vi "Istwerte verarbeiten Regler.vi"(8 "error in (no error)":errorcluster caption="Fehler (Eingang, kein Fehler)", 9 "Index":u16, 10 "Istwerte":u16[](array[numeric]), 11 "mini8 Steuerung PNS Eingang":refnum<class "mini8 Steuerung PNS.lvclass">) -> (0 "error out":errorcluster caption="Fehler (Ausgang)", 3 "mini8 Steuerung PNS Ausgang":refnum<class "mini8 Steuerung PNS.lvclass">)   [LabVIEW 2020, in "mini8 Steuerung PNS.lvclass"]
uses:
  mini8 Steuerung PNS.lvclass
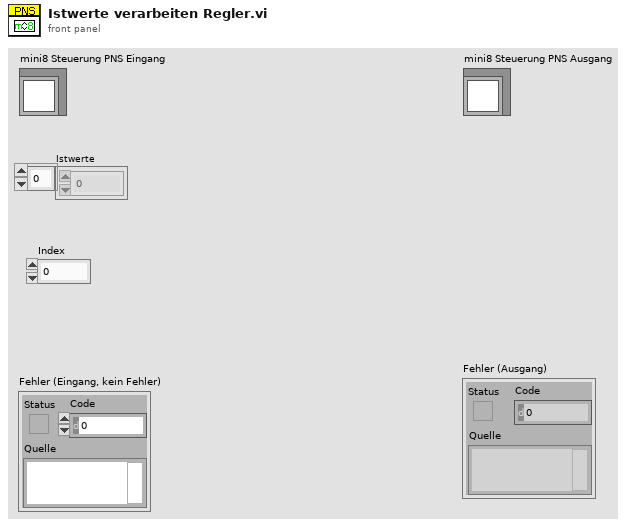
[diagram p1: front panel]
types:
  T1 = typedef "Steuerung PNS.lvclass/Regler.ctl" = cluster{"Istwert":i16, "Sollwert":i16, "Alarm MIN":i16, "Alarm MAX":i16, "Regler sperren":i16, "Analog Ausgang":i16}[]
  T2 = cluster{"Istwerte[0]":u16, "Istwerte[1]":u16, "Istwerte[2]":u16, "Istwerte[3]":u16, "Istwerte[4]":u16, "Istwerte[5]":u16}
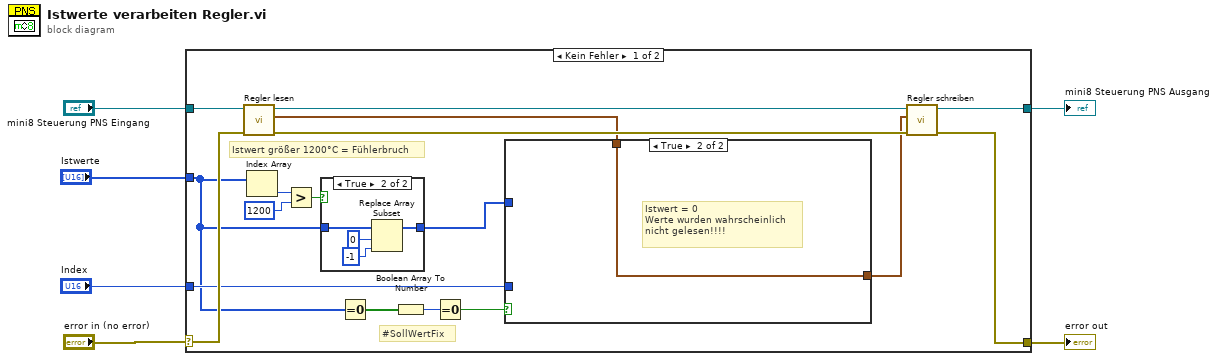
[diagram p0: block diagram]
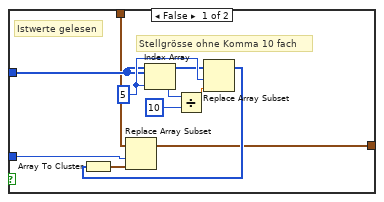
[diagram p2: hidden frame]
diagram:
  n1 = case shown="Kein Fehler" "error in (no error)" {
    selector: "error in (no error)" -> [w15 w41]
    tunnel: [w14 w41] -> w5
    tunnel: [w17 w40] -> w3
    tunnel: "mini8 Steuerung PNS Eingang" -> [w23 w40]
    tunnel: "Istwerte" -> [w9 _]
    tunnel: "Index" -> [w11 _]
    frame No Error {
      # "#SollWertFix"
      # "Istwert größer 1200°C = Fühlerbruch"
      n2 = call-dynamic "Regler lesen.vi"("error in (no error)"=w15, "Steuerung PNS (Eingang)"=w23) -> ("error out"=w16:errorcluster, "Regler"=w12:T1, "Steuerung PNS (Ausgang)"=w18:refnum<class "mini8 Steuerung PNS.lvclass">)  [unwired: 7 in]
      n3 = Index Array(array=w9) -> (element=w20:u16)  [unwired: 1 in]
      n4 = Greater?(x=w20, y=i16 1200) -> (0:w21:bool)
      n5 = case shown="True" w21 {
        tunnel: w9 -> [w35 w36]
        tunnel: [w35 w39] -> w13
        frame False {
        }
        frame True {
          n6 = Replace Array Subset(array=w36, new element=i16 -1 ("Neues Element/Teil-Array"), index=0 ("Index")) -> (w39:u16[])
        }
      }
      n7 = Equal To 0?(x=w9) -> (x = 0?=w8:bool[])
      n8 = Boolean Array To Number(Boolean array=w8) -> (number=w7:u32)
      n9 = Equal To 0?(x=w7) -> (x = 0?=w19:bool)
      n10 = case shown="True" w19 {
        tunnel: w13 -> [w28 _]
        tunnel: w12 -> [w27 w34]
        tunnel: w11 -> [w25 _]
        tunnel: [w24 w34] -> w10
        frame False {
          w33 = 5 ("Index")
          # "Istwerte gelesen"
          # "Stellgrösse ohne Komma 10 fach"
          n11 = Index Array(array=w28, index=w33) -> (element=w32:u16)
          n12 = Divide(x=w32, y=i16 10) -> (x/y=w30:dbl)
          n13 = Replace Array Subset(array=w28, new element=w30, index=w33) -> (w26:u16[])
          n14 = Array To Cluster(array=w26) -> (cluster=w29:T2)
          n15 = Replace Array Subset(array=w27, new element=w29, index=w25) -> (w24:T1)
        }
        frame True {
          # "Istwert = 0\nWerte wurden wahrscheinlich\nnicht gelesen!!!!"
        }
      }
      n16 = call-dynamic "Regler schreiben.vi"("error in (no error)"=w16, "Regler"=w10, "Steuerung PNS (Eingang)"=w18) -> ("error out"=w14:errorcluster, "Steuerung PNS (Ausgang)"=w17:refnum<class "mini8 Steuerung PNS.lvclass">)  [unwired: 7 in]
    }
    frame Error {
    }
  }
  "error out" <- w5
  "mini8 Steuerung PNS Ausgang" <- w3
